vi "post_dust_source.vi"(8 "error in (no error)":errorcluster, 11 "Dust control settings":T1={"Integer Timestamp"=8, "Einzel Voltage"=2.0, "Needle Voltage"=3.0, "Frequency"=4.0, "Width (ms) : 0.1 "=5.0, "Desired Amplitude (V)"=6.0, "X Voltage"=7.0, "Y Voltage"=0.0, "Settings ID"="", "ID#"=0} {"Needle Voltage" min=0.0 max=10.0 step=0.01 format="%.2g"; "Y Voltage" min=0.0 max=9.0 step=0.01 format="%.2g"; "X Voltage" min=0.0 max=9.0 step=0.01 format="%.2g"; "Einzel Voltage" min=0.0 max=10.0 step=0.01 format="%.2g"; "Desired Amplitude (V)" min=0.0 max=10.0 step=0.01 format="%5.2f"; "Width (ms) : 0.1" min=0.05 max=5.0 step=0.01 format="%6.2f"; "Frequency" min=1.0 max=100.0 step=0.01 format="%.1f"}) -> (0 "error out":errorcluster, 3 "Test Server":bool)   [LabVIEW 2013]
uses:
  dust_soruce_control.ctl
  <vilib>/addons/database/NI_Database_API.lvlib
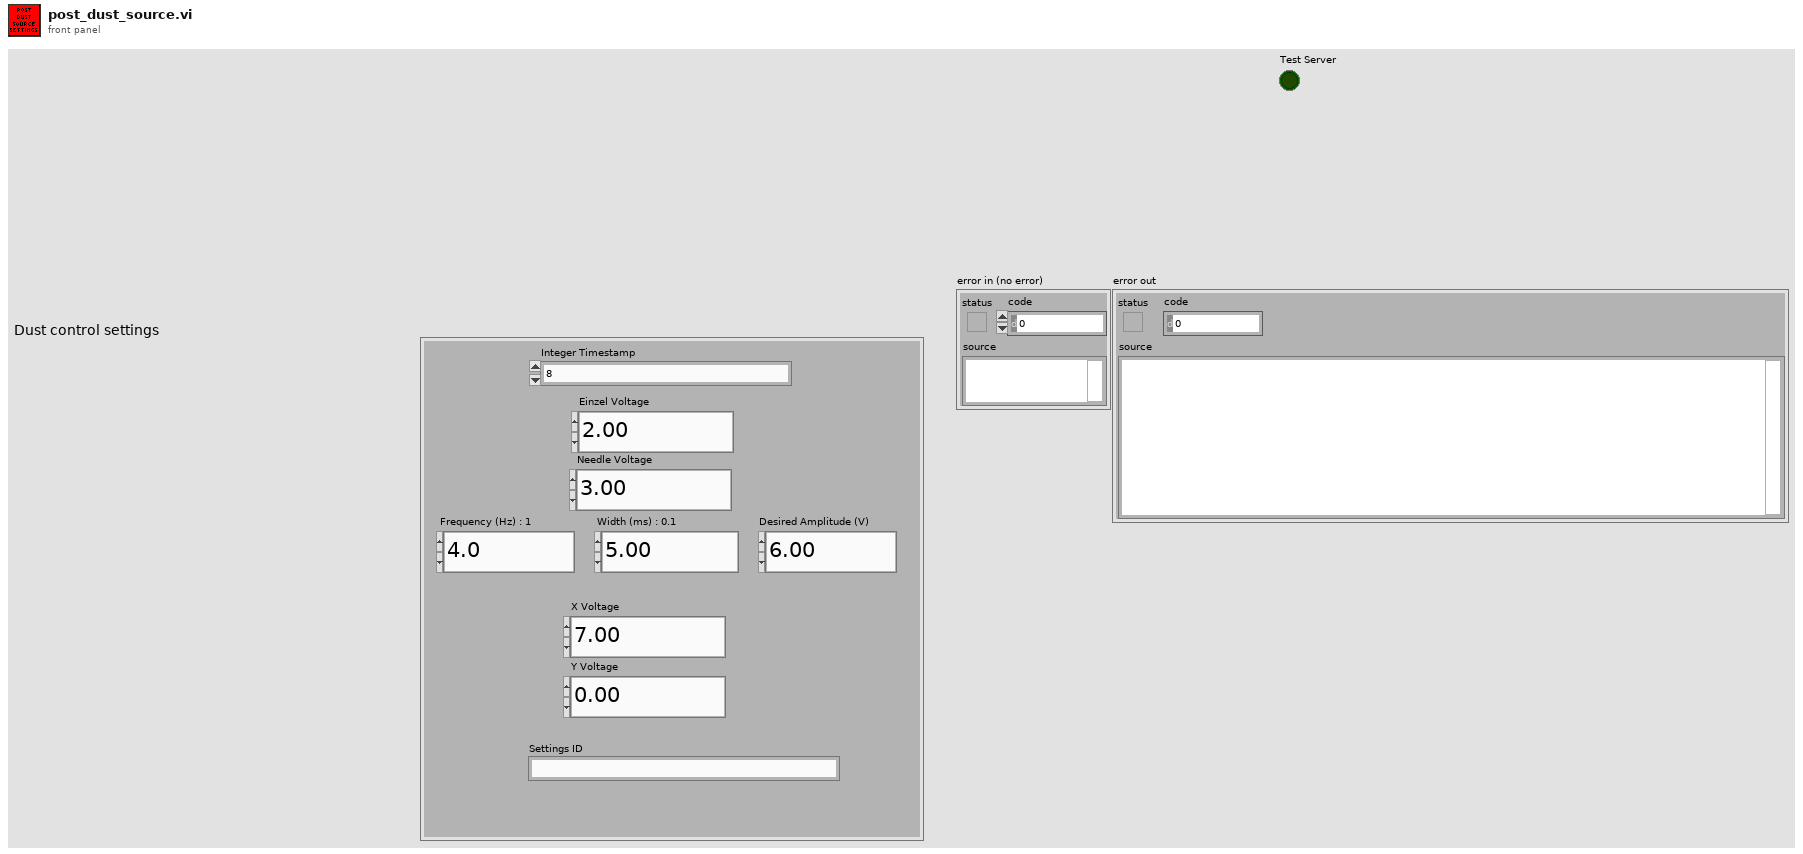
[diagram p1: front panel]
types:
  T1 = typedef "dust_soruce_control.ctl" = cluster{"Integer Timestamp":u64, "Einzel Voltage":dbl, "Needle Voltage":dbl, "Frequency":dbl, "Width (ms) : 0.1 ":dbl, "Desired Amplitude (V)":dbl, "X Voltage":dbl, "Y Voltage":dbl, "Settings ID":string, "ID#":i32}
  T2 = typedef "NI_Database_API.lvlib/Conn ObjectReference.ctl" = refnum<k1>
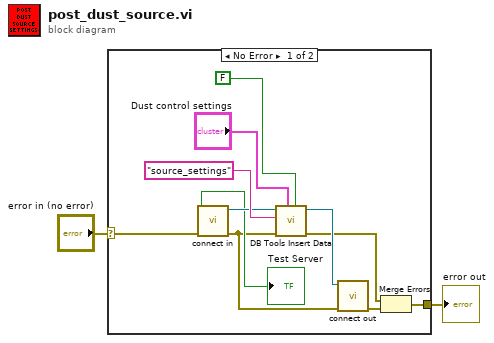
[diagram p0: block diagram]
diagram:
  n1 = case shown="No Error" "error in (no error)" {
    selector: "error in (no error)" -> [w13 w14]
    tunnel: [w3 w14] -> w1
    frame No Error {
      n2 = call "connect in.vi"("error in (no error)"=w13) -> ("error out"=w5:errorcluster, "Database Connection"=w11:T2, "Test Server"=→"Test Server":bool)  [unwired: 6 in]
      n3 = call <vilib>:"DB Tools Insert Data.vi"("create table? (F)"=FALSE, "data"="Dust control settings", "error in (no error)"=w5, "table"="source_settings", "connection reference"=w11) -> ("error out"=w6:errorcluster, "connection reference out"=w10:T2)  [unwired: 5 in]
      n4 = call "connect out.vi"("error in (no error)"=w5, "connection reference"=w10) -> ("error out"=w4:errorcluster)  [unwired: 9 in]
      n5 = Merge Errors(w6, w4) -> (w3:errorcluster)
    }
    frame Error {
    }
  }
  "error out" <- w1
